vi "Exercise2.1-Device Test.vi"() -> ()   [LabVIEW 2013]
uses:
  <instrlib>/rtlsdr/rtlsdr.lvlib
panel:
  out "DevRefnum":u64
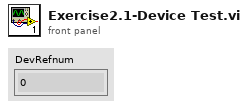
[diagram p1: front panel]
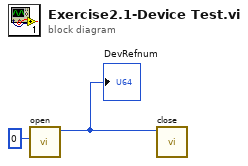
[diagram p0: block diagram]
diagram:
  n1 = call <instrlib>:"open.vi"("index"=u32 0) -> ("DevRefnum"=w1:u64)  [unwired: 9 in, 1 out]
  "DevRefnum" <- w1
  n2 = call <instrlib>:"close.vi"("DevRefnum"=w1) -> ()  [unwired: 9 in, 2 out]
